vi "Write Prompt.vi"(8 "error in (no error)":errorcluster, 10 "Prompt":string, 11 "Report File in":refnum<class "Report File.lvclass">) -> (0 "error out":errorcluster, 3 "Report File out":refnum<class "Report File.lvclass">)   [LabVIEW 2018, in "Report File.lvclass"]
uses:
  Report File.lvclass
  Report File.lvclass/Report File.ctl
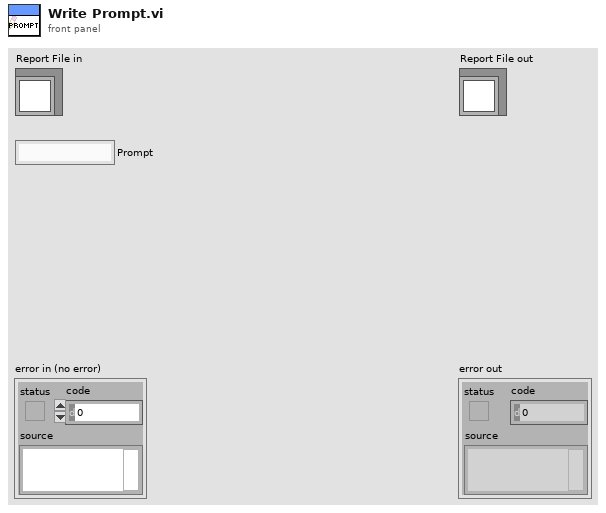
[diagram p1: front panel]
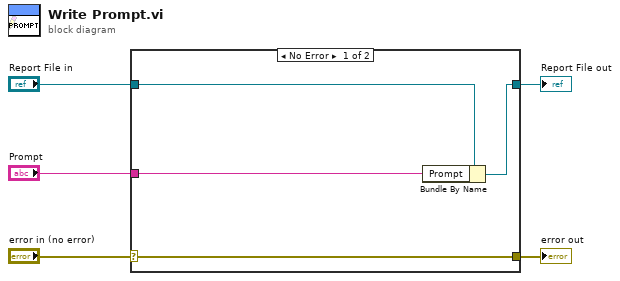
[diagram p0: block diagram]
diagram:
  n1 = case shown="No Error" "error in (no error)" {
    selector: "error in (no error)" -> [w9 w10]
    tunnel: [w9 w10] -> w4
    tunnel: [w7 w11] -> w2
    tunnel: "Report File in" -> [w8 w11]
    tunnel: "Prompt" -> [w6 _]
    frame No Error {
      n2 = Bundle By Name(cluster=w8, "Prompt"=w6) -> (w7:refnum<class "Report File.lvclass">)
    }
    frame Error {
    }
  }
  "error out" <- w4
  "Report File out" <- w2
